vi "Mono camera test.vi"() -> ()   [LabVIEW 2022 SP3]
uses:
  <vilib>/vision/NI_Vision_Development_Module.lvlib
panel:
  out "Loop iterations":i32
  out "Array 2":sgl[](array[numeric])
  out "Array":u8[](array[numeric])
  out "Circles Data (calibrated) (Circle Detection 1)":T1(array[cluster])
  out "Particle Measurements (Pixels) (Data from objects)":dbl[][](array[numeric]) format="%.2f"
  out "Number of Particles (Data from objects)":i32
  out "error out":errorcluster
  in  "Exposure time":dbl(slide) step=100.0 scale=1000.0..10000.0
  out "File-name":path
  out "appended path":path
  in  "stop":bool
  out "Image Out":T2(plugin-control)
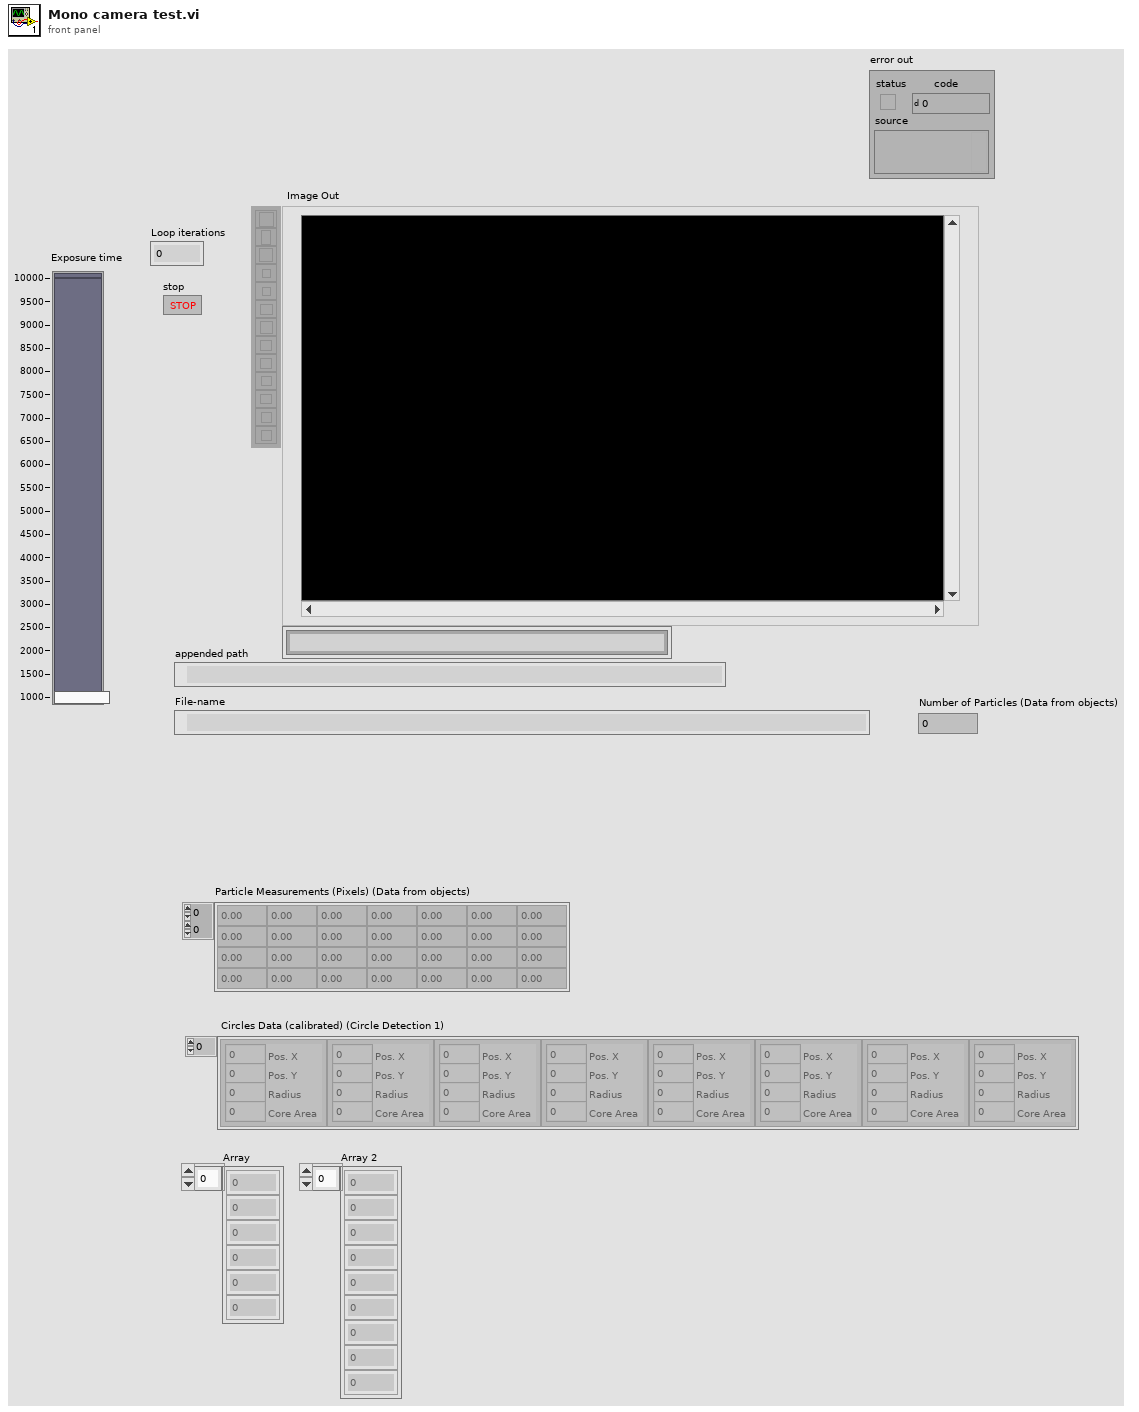
[diagram p1: front panel]
types:
  T1 = cluster{"Pos. X":i32, "Pos. Y":i32, "Radius":i32, "Core Area":i32}[]
  T2 = typedef "IMAQ Image.ctl" = refnum<image>
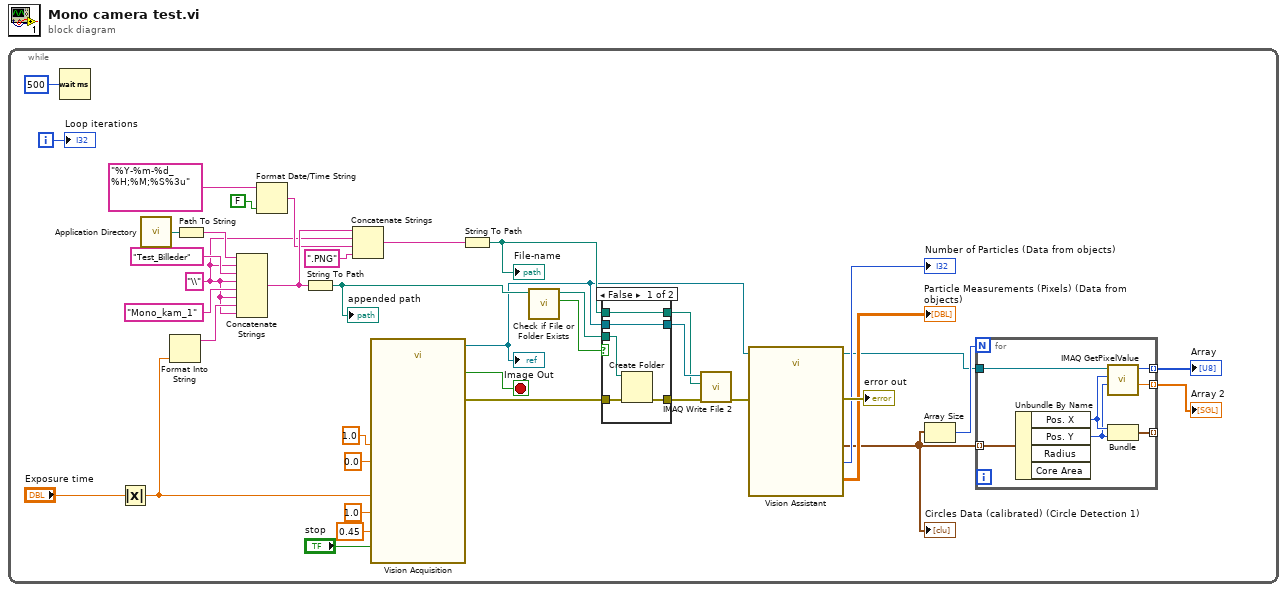
[diagram p0: block diagram]
diagram:
  n1 = while {
    i -> [w10]
    stop <- w11 stop-if-true
    w8 = "\\" ("string")
    n2 = Wait (ms)(milliseconds to wait=u32 500) -> ()  [unwired: 1 out]
    n3 = Absolute Value(x="Exposure time") -> (abs(x)=w5:dbl)
    n4 = call <vilib>:"Application Directory.vi"() -> ("Application Directory"=w35:path)
    n5 = Format Into String(w5) -> (resulting string=w9:string)  [unwired: 3 in, 1 out]
    n6 = Path To String(path=w35) -> (string=w34:string)
    n7 = Concatenate Strings(w34, w8, "Test_Billeder" ("string"), w8, "Mono_kam_1" ("string"), w8, w9, w8) -> (w29:string)
    n8 = Format Date/Time String(time format string (%c)="%Y-%m-%d_%H;%M;%S%3u", UTC format=FALSE) -> (date/time string=w26:string)  [unwired: 1 in]
    n9 = String To Path(string=w29) -> (path=w32:path)
    "appended path" <- w32
    n10 = Concatenate Strings(w29, w8, w26, ".PNG" ("string")) -> (w28:string)
    n11 = call "Vision Acquisition"("AcquisitionFrameRate"=1.0, "ExposureTime"=w5, "Gain"=1.0, "BlackLevel"=0.0, "Gamma"=0.45, "Stop (F)"="stop") -> ("Image Out"=w1:T2, "Stopped"=w11:bool, "error out"=w21:errorcluster)  [unwired: 19 in]
    "Image Out" <- w1
    n12 = String To Path(string=w28) -> (path=w24:path)
    "File-name" <- w24
    n13 = call <vilib>:"Check if File or Folder Exists.vi"("path"=w32) -> ("file or folder exists?"=w30:bool, "dup path"=w31:path)  [unwired: 8 in, 1 out]
    n14 = case shown="False" w30 {
      tunnel: w31 -> [w52 _]
      tunnel: [w51 w55] -> w33
      tunnel: w1 -> [w51 w55]
      tunnel: w24 -> [w50 w54]
      tunnel: [w50 w54] -> w23
      tunnel: w21 -> [w49 w53]
      tunnel: [w48 w53] -> w20
      frame False {
        n15 = Create Folder(path (use dialog)=w52, error in=w49) -> (error out=w48:errorcluster)  [unwired: 1 in, 2 out]
      }
      frame True {
      }
    }
    n16 = call-poly "IMAQ Write File 2"("error in (no error)"=w20, "File Path"=w23, "Image"=w33) -> ("error out"=w19:errorcluster)  [unwired: 7 in, 1 out]
    n17 = call "Vision Assistant"("Image In"=w1, "error in"=w19) -> ("Image Out"=w7:T2, "Circles Data (calibrated) (Circle Detection 1)"=w14:T1, "Number of Particles (Data from objects)"=→"Number of Particles (Data from objects)":i32, "Particle Measurements (Pixels) (Data from objects)"=→"Particle Measurements (Pixels) (Data from objects)":dbl[][], "error out"=→"error out":errorcluster)  [unwired: 20 in, 1 out]
    "Circles Data (calibrated) (Circle Detection 1)" <- w14
    n18 = Array Size(array=w14) -> (size(s)=w15:i32)
    n19 = for {
      N: w15 -> [_]
      tunnel: w14 -> [w47] mode=indexing
      tunnel: [w46] -> w13 mode=indexing
      tunnel: [w43] -> _ mode=indexing
      tunnel: [w42] -> w12 mode=indexing
      tunnel: w7 -> [w41]
      n20 = Unbundle By Name(w47) -> ("Pos. X"=w45:i32, "Pos. Y"=w44:i32)  [unwired: 2 out]
      n21 = call "IMAQ GetPixelValue"("Image"=w41, "X Coordinate"=w45, "Y Coordinate"=w44) -> ("Pixel Value (U8)"=w46:u8, "Pixel Value (Float)"=w42:sgl)  [unwired: 3 in, 3 out]
      n22 = Bundle("Pos. X"=w45, "Pos. Y"=w44) -> (w43:cluster{"Pos. X":i32, "Pos. Y":i32})  [unwired: 1 in]
    }
    "Array" <- w13
    "Array 2" <- w12
    "Loop iterations" <- w10
  }
